vi "ChopStringFromBothSides.vi"(9 "Cut from end":i32, 10 "Cut from start":i32, 11 "String in":string) -> (3 "String out":string)   [LabVIEW 2023]
doc: "Chops off a string from both sides. (begining and end)"
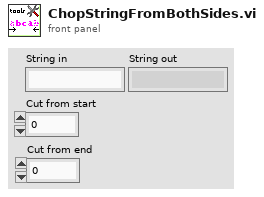
[diagram p1: front panel]
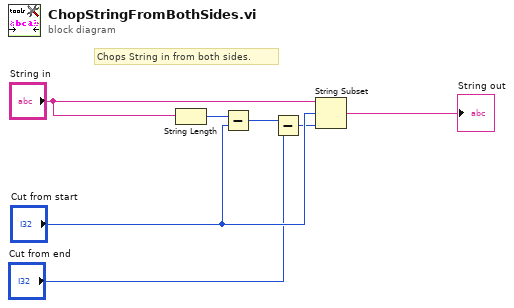
[diagram p0: block diagram]
diagram:
  # "Chops String in from both sides."
  n1 = String Length(string="String in") -> (length=w2:i32)
  n2 = Subtract(x=w2, y="Cut from start") -> (x-y=w4:i32)
  n3 = Subtract(x=w4, y="Cut from end") -> (x-y=w5:i32)
  n4 = String Subset(string="String in", offset (0)="Cut from start", length (rest)=w5) -> (substring=→"String out":string)
